vi "Example Create JSON Schema.vi"() -> ()   [LabVIEW 2023]
uses:
  Unit Tests/Support/Test Enum 2--enum.ctl
  7dc4fba5-8a80-492e-b267-0080a53f7d5c.vi
  <vilib>/JDP Science/JSONtext/Variant to JSON Text.vi
  <vilib>/JDP Science/JSONtext/LVClass Serializer/JSONtext LVClass Serializer.lvclass
  <vilib>/JDP Science/JSONtext/JSONtext.lvlib
  JSON Schema Generator.lvlib
panel:
  in  "Cluster":cluster{"Test Enum 2":T1}
  out "error out":errorcluster
  out "<JSON>":string
  in  "Example Cluster":T2={"ProductId"=1, "productName"="A green door", "price"=12.5, "tags"=["home", "green"], "ProductNumber"=1, "ProductInfoInternal"={"ProductState"=enum."Active", "State Info"={"Date"="", "Time"=0.0}, "Test Enum"=enum."Select 1"}, "Product History"=[], "Test Enum 2"=enum."Select 1"}
  out "Valid?":bool
  in  "Description":string
  in  "Title":string="test"
  out "JSON Schema out":string caption="JSON Schema"
  # "Example"
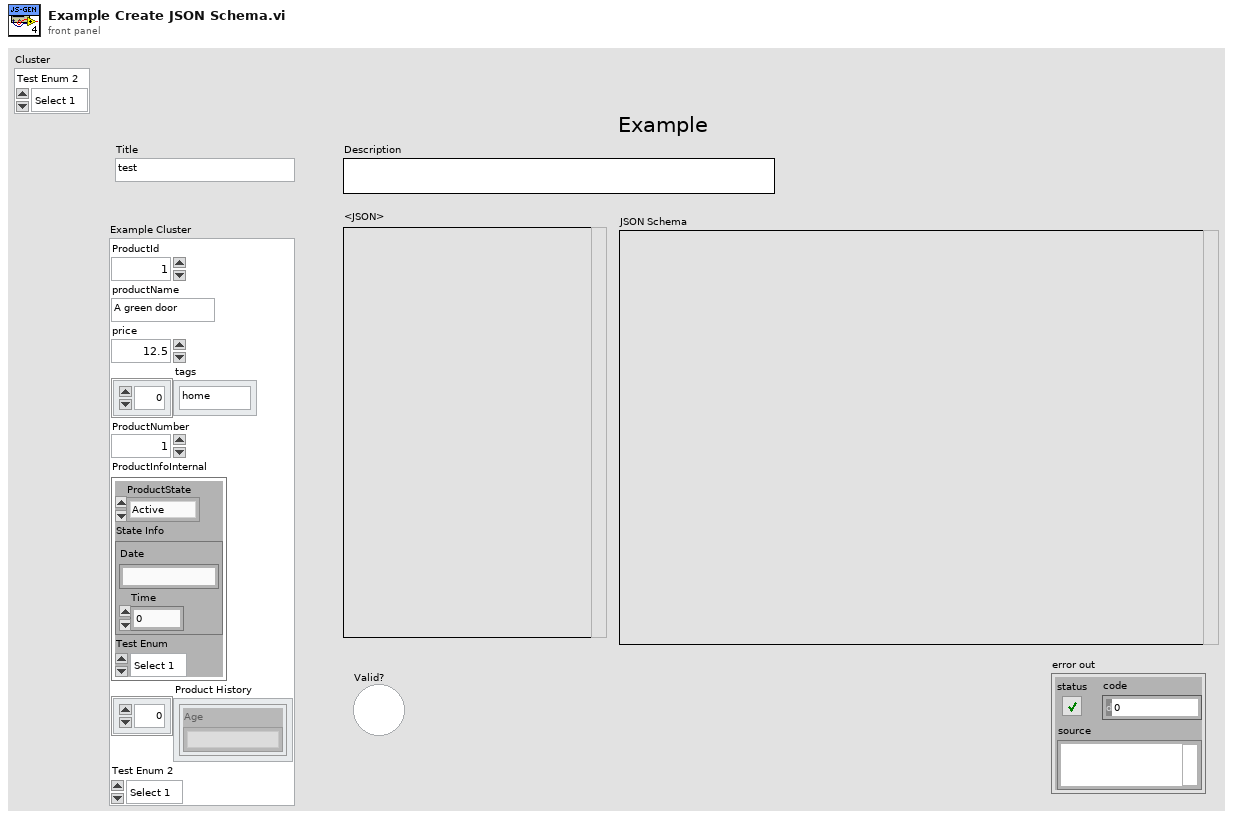
[diagram p1: front panel]
types:
  T1 = typedef "Test Enum 2--enum.ctl" = enum16{"Select 1", "Select 2"}
  T2 = cluster{"ProductId":i32, "productName":string, "price":dbl, "tags":string[], "ProductNumber":i32, "ProductInfoInternal":cluster{"ProductState":enum16{"Active", "InActive"}, "State Info":cluster{"Date":string, "Time":dbl}, "Test Enum":T1}, "Product History":cluster{"Age":string}[], "Test Enum 2":T1}
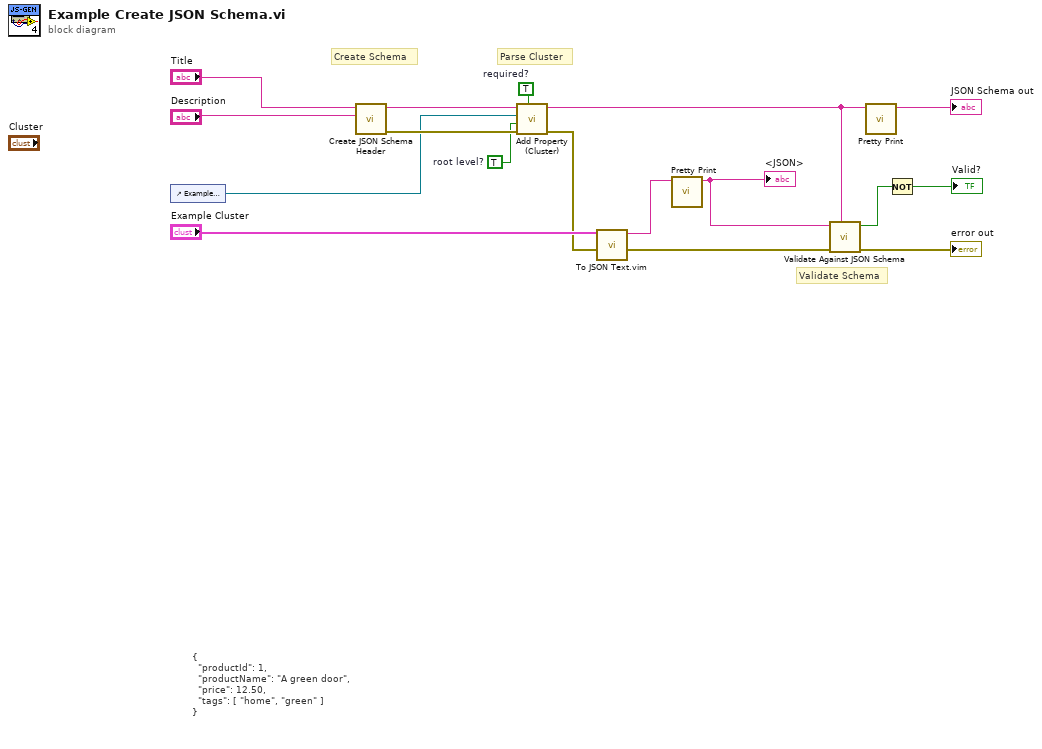
[diagram p0: block diagram]
diagram:
  w6 = TRUE  # required?
  w8 = TRUE  # root level?
  # "Validate Schema"
  # "Parse Cluster"
  # "Create Schema"
  # "{\n  \"productId\": 1,\n  \"productName\": \"A green door\",\n  \"price\": 12.50,\n  \"tags\": [ \"home\", \"green\" ]\n}"
  n1 = control-ref of="Example Cluster"() -> (w5:refnum<vi>)
  n2 = call "Create JSON Schema Header.vi"("Description"="Description", "Title"="Title") -> ("error out"=w11:errorcluster, "JSON Schema out"=w13:string)  [unwired: 8 in]
  n3 = call "Add Property (Cluster).vi"("required?"=w6, "error in (no error)"=w11, "root level? (false)"=w8, "Cluster in"=w5, "JSON Schema in"=w13) -> ("error out"=w3:errorcluster, "JSON Schema out"=w12:string)  [unwired: 5 in]
  n4 = call "To JSON Text.vim"("error in (no error)"=w3, "Anything"="Example Cluster") -> ("error out"=w2:errorcluster, "<JSON>"=w10:string)  [unwired: 8 in]
  n5 = call <vilib>:"Pretty Print.vi"("JSON"=w10) -> ("<JSON>"=w9:string)  [unwired: 8 in, 2 out]
  "<JSON>" <- w9
  n6 = call <vilib>:"Validate Against JSON Schema.vi"("JSON Schema"=w12, "error in (no error)"=w2, "JSON"=w9) -> ("error out"=→"error out":errorcluster, "Invalid"=w14:bool)  [unwired: 4 in, 3 out]
  n7 = call <vilib>:"Pretty Print.vi"("JSON"=w12) -> ("<JSON>"=→"JSON Schema out":string)  [unwired: 8 in, 2 out]
  n8 = Not(x=w14) -> (.not. x?=→"Valid?":bool)
